vi "Test2.vi"() -> ()   [LabVIEW 2012]
uses:
  <vilib>/Rock Robotics/SystemInterfaces/DIO/FPGA_DIOPWMChannel.ctl
  <vilib>/Rock Robotics/WPI/SafetyOutput/WPI_SafetyOutputConfigMenu.ctl
  <vilib>/Rock Robotics/SystemInterfaces/Typedef/FPGA_TypedefDigitalModule.ctl
  <vilib>/Rock Robotics/SystemInterfaces/DIO/FPGA_DIOChannel.ctl
  <vilib>/Rock Robotics/WPI/Encoder/WPI_EncoderType.ctl
  <vilib>/Rock Robotics/WPI/RobotDrive/WPI_RobotDriveOpen2MotorWithTalon.vi
  <vilib>/Rock Robotics/WPI/Counter/WPI_CounterDigitalInputToDigitalSource.vi
  <vilib>/addons/control/pid/pid.llb/PID (DBL).vi
  <vilib>/Rock Robotics/WPI/RobotDrive/WPI_RobotDriveGetSetRefNum.vi
  <vilib>/addons/control/pid/NI_PID_pid.lvlib
panel:
  in  "stop":bool
  out "Posistioned":string="Nothing"
  in  "Angle Target":dbl
  in  "Distance From Target":dbl
  out "Current Status":string="Roaming"
  # "Check that the robot moves the specified angle and distance. The gear ratio of the wheels\nwill need to be added into both this and the final code. Also this code will keep repeating,\nbut the robot should only move once (Because we don't reset the encoders). If the robot \nmoves more than once, the thresholds for it finishing need to be changed."
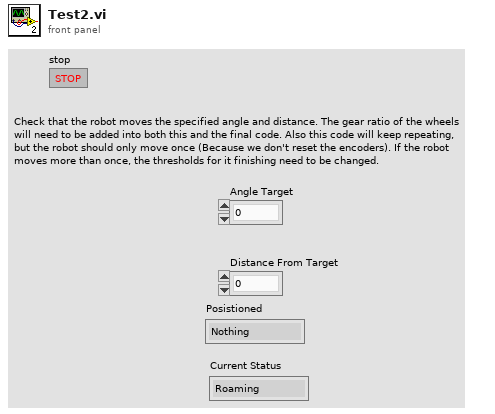
[diagram p1: front panel]
types:
  T1 = typedef "WPI_EncoderType.ctl" = enum16{"1x", "2x", "4x"}
  T2 = typedef "FPGA_DIOChannel.ctl" = enum8{"DIO 1", "DIO 2", "DIO 3", "DIO 4", "DIO 5", "DIO 6", "DIO 7", "DIO 8", "DIO 9", "DIO 10", "DIO 11", "DIO 12", "DIO 13", "DIO 14", "Invalid"}
  T3 = typedef "WPI_SafetyOutputConfigMenu.ctl" = enum16{"Enable", "Disable"}
  T4 = cluster{"proportional gain (Kc)":dbl, "integral time (Ti, min)":dbl, "derivative time (Td, min)":dbl}
  T5 = typedef "FPGA_TypedefDigitalModule.ctl" = enum16{"Digital Module 1", "Digital Module 2"}
  T6 = typedef "FPGA_DIOPWMChannel.ctl" = enum8{"PWM 1", "PWM 2", "PWM 3", "PWM 4", "PWM 5", "PWM 6", "PWM 7", "PWM 8", "PWM 9", "PWM 10", "Invalid"}
  T7 = typedef "WPI_DigitalInputDevRef.ctl" = cluster{"DevStatus":errorcluster, "DIO Channel":T2, "Digital Module":T5}
  T8 = typedef "FPGA_CounterEncoderSourceConvertionLVSourceType.ctl" = cluster{"DevStatus":errorcluster, "AnalogTriggerMode?":bool, "DigitalMode":cluster{"Digital Module":T5, "DIO Channel":T9}, "AnalogTriggerMode":cluster{"AnalogTriggerIndex":T10, "OutputType":T11}}
  T9 = typedef "FPGA_DIODigitalSourceChannel.ctl" = enum8{"DIO 1", "DIO 2", "DIO 3", "DIO 4", "DIO 5", "DIO 6", "DIO 7", "DIO 8", "DIO 9", "DIO 10", "DIO 11", "DIO 12", "DIO 13", "DIO 14", "Disabled"}
  T10 = typedef "FPGA_AnalogTriggerIndex.ctl" = enum8{"Trig 0", "Trig 1", "Trig 2", "Trig 3", "Trig 4", "Trig 5", "Trig 6", "Trig 7", "Invalid"}
  T11 = typedef "FPGA_AnalogTriggerOutType.ctl" = enum16{"InWindow", "TriggerState", "Rising", "Falling"}
  T12 = typedef "WPI_EncoderDevRef.ctl" = cluster{"DevStatus":errorcluster, "EncoderIndex":T13, "CounterIndex":T14, "DistancePerCount":dbl, "Decoding Type":T1}
  T13 = typedef "FPGA_EncoderIdx.ctl" = enum8{"Enc 0", "Enc 1", "Enc 2", "Enc 3", "Invalid"}
  T14 = typedef "FPGA_CounterCtrSystemIndex.ctl" = enum8{"Ctr 0", "Ctr 1", "Ctr 2", "Ctr 3", "Ctr 4", "Ctr 5", "Ctr 6", "Ctr 7", "Invalid"}
  T15 = typedef "WPI_RobotDriveDevRef.ctl" = cluster{"DevStatus":errorcluster, "Motors[]":T16[], "Square Inputs":bool, "Max Output":dbl, "Isochronous":bool}
  T16 = typedef "WPI_MotorControlDeviceRef.ctl" = cluster{"DeviceStatus":errorcluster, "Type":enum16{"PWM", "CAN"}, "PWM":cluster{"Digital Module":T5, "PWM Channel":T6, "DeadBand":T17}, "CAN":cluster{"Device Number":u8, "Control Mode":T18, "Semaphore":T19, "Max Vout":dbl}, "Invert":bool, "TransformRef":T20, "InvTransformRef":T20}
  T17 = typedef "WPI_PWMDeadband.ctl" = cluster{"Name":string, "maxPositivePwm":i32, "minPositivePwm":i32, "centerPwm":i32, "maxNegativePwm":i32, "minNegativePwm":i32, "angularRange":u16}
  T18 = typedef "WPI_CANJaguar_ControlMode.ctl" = enum8{"Percent VBus", "Current", "Speed", "Position", "Voltage"}
  T19 = typedef "Semaphore RefNum" = refnum<k1>
  T20 = typedef "WPI_PWMTransform_ConPane.ctl" = refnum<vi>
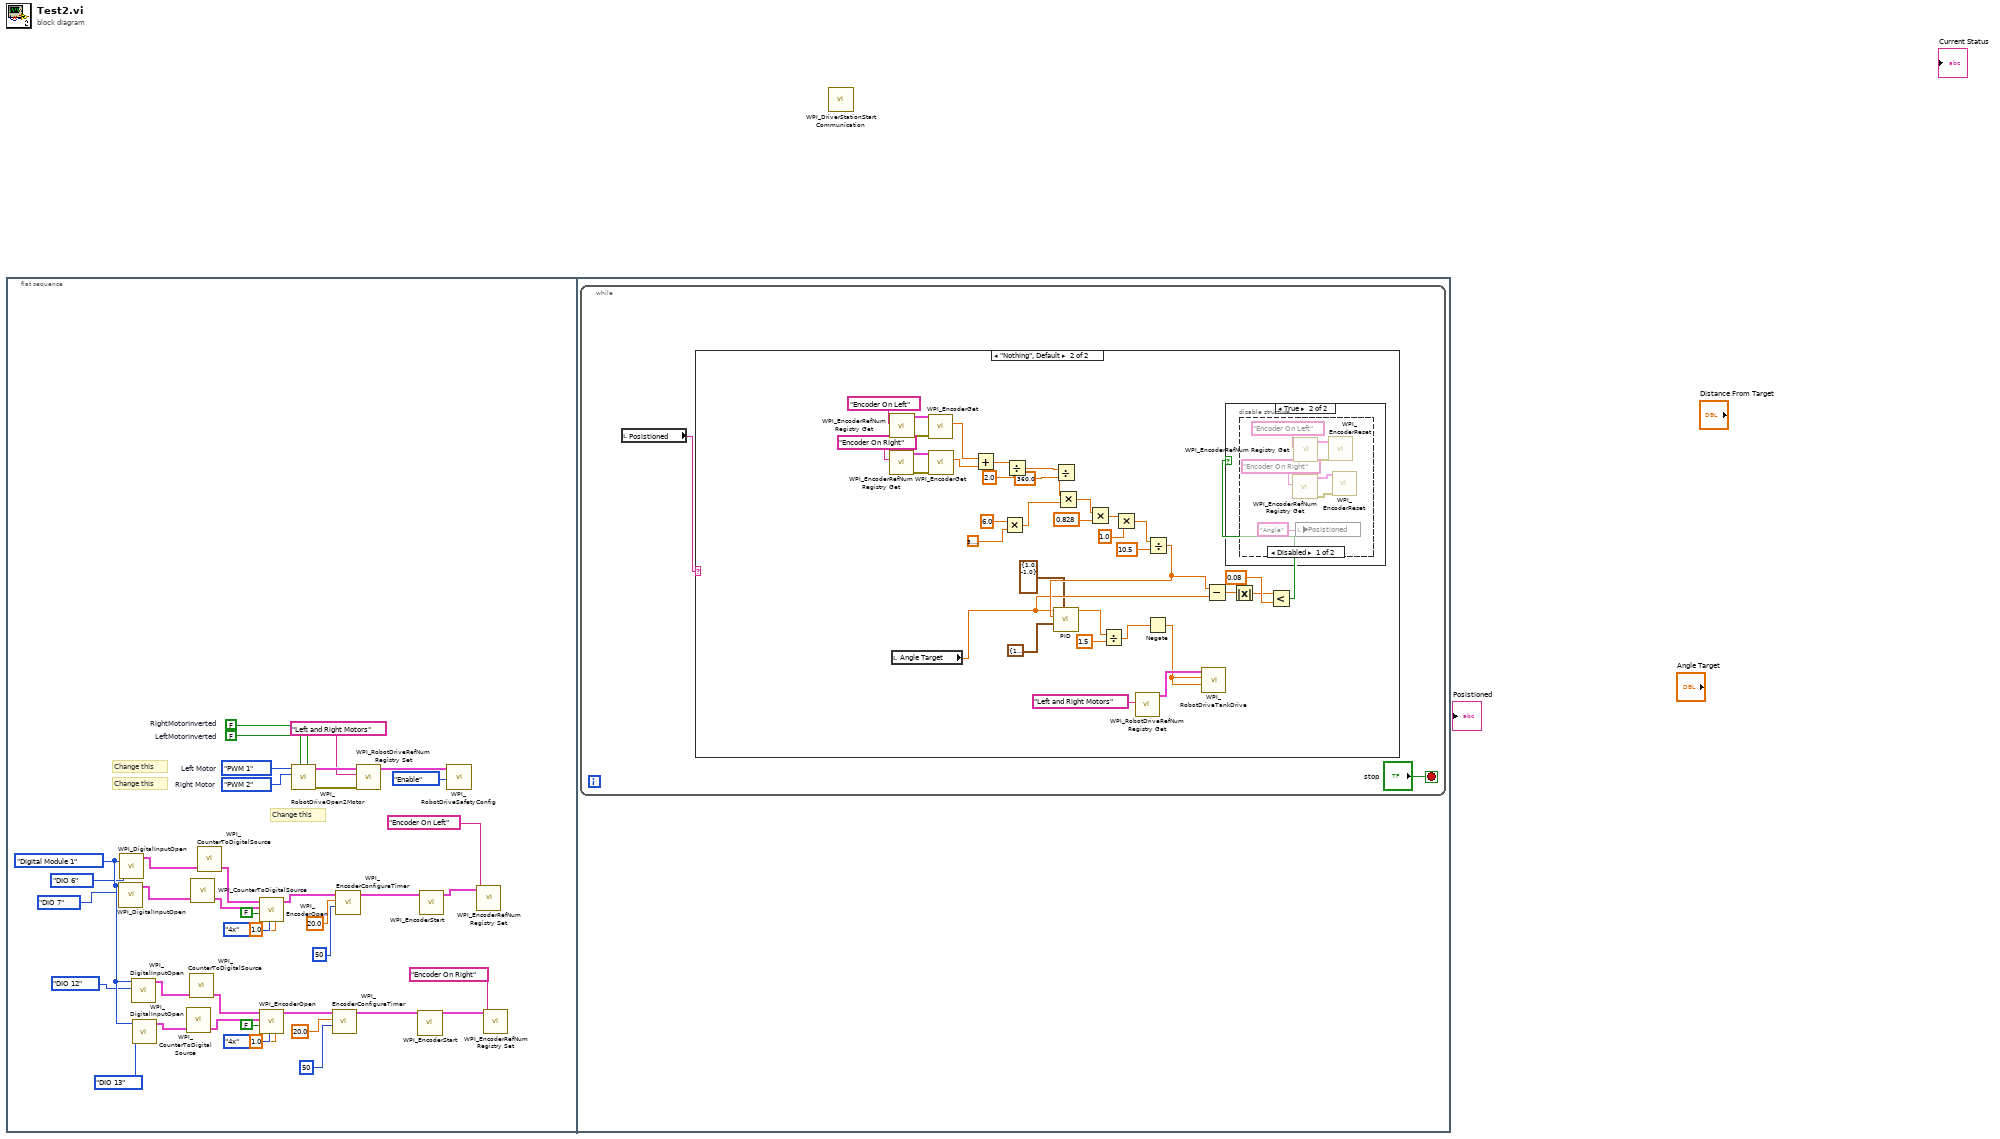
[diagram p0: block diagram]
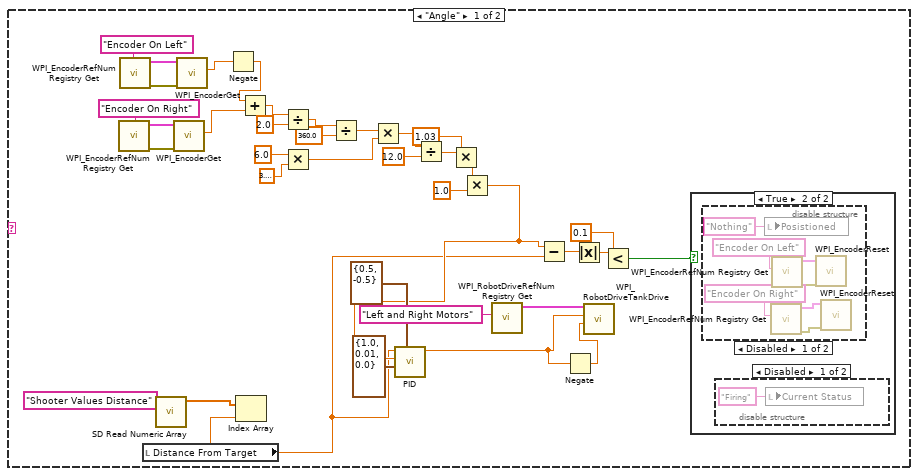
[diagram p2: hidden frame]
diagram:
  n1 = flat-sequence {
    frame #0 {
      w31 = FPGA_TypedefDigitalModule."Digital Module 1" ("Digital Module (Module 1)")
      w34 = FPGA_DIOPWMChannel."PWM 2"  # Right Motor
      w35 = FPGA_DIOPWMChannel."PWM 1"  # Left Motor
      w39 = FALSE  # LeftMotorInverted
      w40 = FALSE  # RightMotorInverted
      # "Change this"
      # "Change this"
      # "Change this"
      n2 = call <vilib>:"WPI_DigitalInputOpen.vi"("DIO Channel"=FPGA_DIOChannel."DIO 7", "Digital Module (Module 1)"=w31) -> ("DigitalInputDevRef"=w24:T7)  [unwired: 8 in, 1 out]
      n3 = call <vilib>:"WPI_DigitalInputOpen.vi"("DIO Channel"=FPGA_DIOChannel."DIO 6", "Digital Module (Module 1)"=w31) -> ("DigitalInputDevRef"=w23:T7)  [unwired: 8 in, 1 out]
      n4 = call <vilib>:"WPI_DigitalInputOpen.vi"("DIO Channel"=FPGA_DIOChannel."DIO 12", "Digital Module (Module 1)"=w31) -> ("DigitalInputDevRef"=w25:T7)  [unwired: 8 in, 1 out]
      n5 = call <vilib>:"WPI_DigitalInputOpen.vi"("DIO Channel"=FPGA_DIOChannel."DIO 13", "Digital Module (Module 1)"=w31) -> ("DigitalInputDevRef"=w26:T7)  [unwired: 8 in, 1 out]
      n6 = call-poly <vilib>:"WPI_CounterToDigitalSource.vi"("DigitalInputDevRef"=w26) -> ("Digital Source"=w19:T8)  [unwired: 6 in]
      n7 = call-poly <vilib>:"WPI_CounterToDigitalSource.vi"("DigitalInputDevRef"=w25) -> ("Digital Source"=w20:T8)  [unwired: 6 in]
      n8 = call-poly <vilib>:"WPI_CounterToDigitalSource.vi"("DigitalInputDevRef"=w24) -> ("Digital Source"=w21:T8)  [unwired: 6 in]
      n9 = call-poly <vilib>:"WPI_CounterToDigitalSource.vi"("DigitalInputDevRef"=w23) -> ("Digital Source"=w22:T8)  [unwired: 6 in]
      n10 = call <vilib>:"WPI_EncoderOpen.vi"("DistancePerCount"=1.0, "Decoding Type"=WPI_EncoderType."4x", "Invert Direction (False)"=FALSE, "BSource"=w21, "ASource"=w22) -> ("EncoderDevRef"=w18:T12)  [unwired: 5 in, 1 out]
      n11 = call <vilib>:"WPI_EncoderOpen.vi"("DistancePerCount"=1.0, "Decoding Type"=WPI_EncoderType."4x", "Invert Direction (False)"=FALSE, "BSource"=w19, "ASource"=w20) -> ("EncoderDevRef"=w17:T12)  [unwired: 5 in, 1 out]
      n12 = call-poly <vilib>:"WPI_RobotDriveOpen2Motor.vi"("Right Motor Inverted"=w40, "Left Motor Inverted"=w39, "Right Motor"=w34, "Left Motor"=w35) -> ("error out"=w36:errorcluster, "RobotDriveDevRef"=w38:T15)  [unwired: 1 in, 5 out]
      n13 = call <vilib>:"WPI_EncoderConfigureTimer.vi"("Number Samples to Average"=u8 50, "Minimum Rate"=20.0, "EncoderDevRef"=w17) -> ("EncoderDevRef"=w15:T12)  [unwired: 7 in, 1 out]
      n14 = call <vilib>:"WPI_EncoderConfigureTimer.vi"("Number Samples to Average"=u8 50, "Minimum Rate"=20.0, "EncoderDevRef"=w18) -> ("EncoderDevRef"=w16:T12)  [unwired: 7 in, 1 out]
      n15 = call <vilib>:"WPI_RobotDriveRefNum Registry Set.vi"("error in (no error)"=w36, "refnum name"="Left and Right Motors", "RobotDriveDevRef"=w38) -> ("RobotDriveDevRef"=w33:T15)  [unwired: 8 out]
      n16 = call <vilib>:"WPI_EncoderStart.vi"("EncoderDevRef"=w15) -> ("EncoderDevRef"=w14:T12)  [unwired: 9 in, 1 out]
      n17 = call <vilib>:"WPI_EncoderStart.vi"("EncoderDevRef"=w16) -> ("EncoderDevRef"=w13:T12)  [unwired: 9 in, 1 out]
      n18 = call <vilib>:"WPI_RobotDriveSafetyConfig.vi"("mode"=WPI_SafetyOutputConfigMenu."Enable", "RobotDriveDevRef"=w33) -> ()  [unwired: 8 in, 2 out]
      n19 = call <vilib>:"WPI_EncoderRefNum Registry Set.vi"("refnum name"="Encoder On Left", "EncoderDevRef"=w13) -> ()  [unwired: 8 in, 2 out]
      n20 = call <vilib>:"WPI_EncoderRefNum Registry Set.vi"("refnum name"="Encoder On Right", "EncoderDevRef"=w14) -> ()  [unwired: 8 in, 2 out]
    }
    frame #1 {
      n21 = while {
        stop <- "stop" stop-if-true
        n22 = local read "Posistioned"() -> (w42:string)
        n23 = case shown="\"Nothing\", Default" w42 {
          frame "Angle" {
            n24 = call <vilib>:"WPI_EncoderRefNum Registry Get.vi"("refnum name"="Encoder On Right") -> ("error out"=w56:errorcluster, "EncoderDevRef"=w57:T12)  [unwired: 9 in]
            n25 = call <vilib>:"WPI_EncoderRefNum Registry Get.vi"("refnum name"="Encoder On Left") -> ("error out"=w54:errorcluster, "EncoderDevRef"=w55:T12)  [unwired: 9 in]
            n26 = local read "Distance From Target"() -> (w43:dbl)
            n27 = call <vilib>:"SD Read Numeric Array.vi"("Name"="Shooter Values Distance") -> ("Numeric Array"=w74:dbl[])  [unwired: 8 in, 2 out]
            n28 = call <vilib>:"WPI_EncoderGet.vi"("error in (no error)"=w56, "EncoderDevRef"=w57) -> ("Distance"=w60:dbl)  [unwired: 4 in, 5 out]
            n29 = call <vilib>:"WPI_EncoderGet.vi"("error in (no error)"=w54, "EncoderDevRef"=w55) -> ("Distance"=w46:dbl)  [unwired: 4 in, 5 out]
            n30 = Negate(x=w46) -> (-x=w45:dbl)
            n31 = Index Array(array=w74, index=w43) -> ()  [unwired: 1 out]
            n32 = Add(x=w45, y=w60) -> (x+y=w61:dbl)
            n33 = Divide(x=w61, y=2.0) -> (x/y=w65:dbl)
            n34 = Multiply(x=6.0, y=3.141592653589793) -> (x*y=w68:dbl)
            n35 = Divide(x=w65, y=360.0) -> (x/y=w67:dbl)
            n36 = Multiply(x=w67, y=w68) -> (x*y=w69:dbl)
            n37 = Divide(x=w69, y=12.0) -> (x/y=w50:dbl)
            n38 = Multiply(x=w50, y=1.03) -> (x*y=w48:dbl)
            n39 = Multiply(x=w48, y=1.0) -> (x*y=w44:dbl)
            n40 = call-poly <vilib>:"PID.vi"("output range"=cluster{"output high":dbl, "output low":dbl} {"output high"=0.5, "output low"=-0.5}, "PID gains"=T4 {"proportional gain (Kc)"=1.0, "integral time (Ti, min)"=0.01, "derivative time (Td, min)"=0.0}, "process variable"=w44, "setpoint"=w43) -> ("output"=w51:dbl)  [unwired: 6 in, 1 out]
            n41 = call <vilib>:"WPI_RobotDriveRefNum Registry Get.vi"("refnum name"="Left and Right Motors") -> ("RobotDriveDevRef"=w72:T15)  [unwired: 9 in, 1 out]
            n42 = Subtract(x=w44, y=w43) -> (x-y=w76:dbl)
            n43 = Negate(x=w51) -> (-x=w53:dbl)
            n44 = Absolute Value(x=w76) -> (abs(x)=w77:dbl)
            n45 = call <vilib>:"WPI_RobotDriveTankDrive.vi"("Right axis value"=w53, "Left axis value"=w51, "RobotDriveDevRef"=w72) -> ()  [unwired: 6 in, 3 out]
            n46 = Less?(x=w77, y=0.1) -> (x < y?=w79:bool)
            n47 = case shown="True" w79 {
              frame False {
              }
              frame True {
                n48 = disable-structure shown="Disabled" {
                  frame Disabled {
                    n49 = local write "Posistioned"("Nothing" ("Posistioned")) -> ()
                    n50 = call <vilib>:"WPI_EncoderRefNum Registry Get.vi"("refnum name"="Encoder On Right") -> ("error out"=w84:errorcluster, "EncoderDevRef"=w85:T12)  [unwired: 9 in]
                    n51 = call <vilib>:"WPI_EncoderRefNum Registry Get.vi"("refnum name"="Encoder On Left") -> ("error out"=w82:errorcluster, "EncoderDevRef"=w83:T12)  [unwired: 9 in]
                    n52 = call <vilib>:"WPI_EncoderReset.vi"("error in (no error)"=w82, "EncoderDevRef"=w83) -> ()  [unwired: 8 in, 2 out]
                    n53 = call <vilib>:"WPI_EncoderReset.vi"("error in (no error)"=w84, "EncoderDevRef"=w85) -> ()  [unwired: 8 in, 2 out]
                  }
                  frame Enabled {
                  }
                }
                n54 = disable-structure shown="Disabled" {
                  frame Disabled {
                    n55 = local write "Current Status"("Firing" ("Current Status")) -> ()
                  }
                  frame Enabled {
                  }
                }
              }
            }
          }
          frame "Nothing", Default {
            n56 = call <vilib>:"WPI_EncoderRefNum Registry Get.vi"("refnum name"="Encoder On Right") -> ("error out"=w121:errorcluster, "EncoderDevRef"=w120:T12)  [unwired: 9 in]
            n57 = call <vilib>:"WPI_EncoderRefNum Registry Get.vi"("refnum name"="Encoder On Left") -> ("error out"=w123:errorcluster, "EncoderDevRef"=w122:T12)  [unwired: 9 in]
            n58 = local read "Angle Target"() -> (w99:dbl)
            n59 = call <vilib>:"WPI_EncoderGet.vi"("error in (no error)"=w123, "EncoderDevRef"=w122) -> ("Distance"=w117:dbl)  [unwired: 4 in, 5 out]
            n60 = call <vilib>:"WPI_EncoderGet.vi"("error in (no error)"=w121, "EncoderDevRef"=w120) -> ("Distance"=w97:dbl)  [unwired: 4 in, 5 out]
            n61 = Add(x=w117, y=w97) -> (x+y=w116:dbl)
            n62 = Multiply(x=6.0, y=3.141592653589793) -> (x*y=w110:dbl)
            n63 = Divide(x=w116, y=2.0) -> (x/y=w112:dbl)
            n64 = Divide(x=w112, y=360.0) -> (x/y=w104:dbl)
            n65 = Multiply(x=w104, y=w110) -> (x*y=w92:dbl)
            n66 = Multiply(x=w92, y=0.828) -> (x*y=w90:dbl)
            n67 = Multiply(x=w90, y=1.0) -> (x*y=w89:dbl)
            n68 = call <vilib>:"WPI_RobotDriveRefNum Registry Get.vi"("refnum name"="Left and Right Motors") -> ("RobotDriveDevRef"=w106:T15)  [unwired: 9 in, 1 out]
            n69 = Divide(x=w89, y=10.5) -> (x/y=w100:dbl)
            n70 = call-poly <vilib>:"PID.vi"("output range"=cluster{"output high":dbl, "output low":dbl} {"output high"=1.0, "output low"=-1.0}, "PID gains"=T4 {"proportional gain (Kc)"=1.0, "integral time (Ti, min)"=0.01, "derivative time (Td, min)"=0.0}, "process variable"=w100, "setpoint"=w99) -> ("output"=w105:dbl)  [unwired: 6 in, 1 out]
            n71 = Divide(x=w105, y=1.5) -> (x/y=w96:dbl)
            n72 = Negate(x=w96) -> (-x=w95:dbl)
            n73 = call <vilib>:"WPI_RobotDriveTankDrive.vi"("Right axis value"=w95, "Left axis value"=w95, "RobotDriveDevRef"=w106) -> ()  [unwired: 6 in, 3 out]
            n74 = Subtract(x=w100, y=w99) -> (x-y=w101:dbl)
            n75 = Absolute Value(x=w101) -> (abs(x)=w102:dbl)
            n76 = Less?(x=w102, y=0.08) -> (x < y?=w94:bool)
            n77 = case shown="True" w94 {
              frame False {
              }
              frame True {
                n78 = disable-structure shown="Disabled" {
                  frame Disabled {
                    n79 = call <vilib>:"WPI_EncoderRefNum Registry Get.vi"("refnum name"="Encoder On Right") -> ("error out"=w126:errorcluster, "EncoderDevRef"=w125:T12)  [unwired: 9 in]
                    n80 = call <vilib>:"WPI_EncoderRefNum Registry Get.vi"("refnum name"="Encoder On Left") -> ("error out"=w128:errorcluster, "EncoderDevRef"=w127:T12)  [unwired: 9 in]
                    n81 = local write "Posistioned"("Angle" ("Posistioned")) -> ()
                    n82 = call <vilib>:"WPI_EncoderReset.vi"("error in (no error)"=w128, "EncoderDevRef"=w127) -> ()  [unwired: 8 in, 2 out]
                    n83 = call <vilib>:"WPI_EncoderReset.vi"("error in (no error)"=w126, "EncoderDevRef"=w125) -> ()  [unwired: 8 in, 2 out]
                  }
                  frame Enabled {
                  }
                }
              }
            }
          }
        }
      }
    }
  }
  n84 = call <vilib>:"WPI_DriverStationStart Communication.vi"() -> ()  [unwired: 12 in]
